vi "emi_FP Show.vi"(5 "VI Refnum(This vi)":refnum<vi>, 7 "Show time s(0)":dbl, 9 "error in (no error)":errorcluster) -> (6 "VI Refnum":refnum<vi>, 10 "error out":errorcluster)   [LabVIEW 2011]
doc: "If Front panel not open, opens it\nFades in 'vi to tarnsparensy = 0%\nUses time instead of number of iterations to avoid overly long fade ins when processing power is at a premium.\ns\nIf no VI ref in, then the VI containing this VI is used.\nIf VI has multiple panes, only the first pane will be used.\n\nOn error in: Does not run."
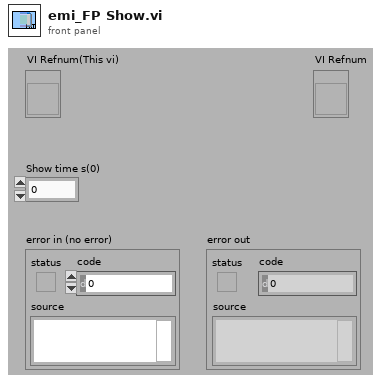
[diagram p1: front panel]
types:
  T1 = enum32{"Invalid", "Standard", "Closed", "Hidden", "Minimized", "Maximized"}
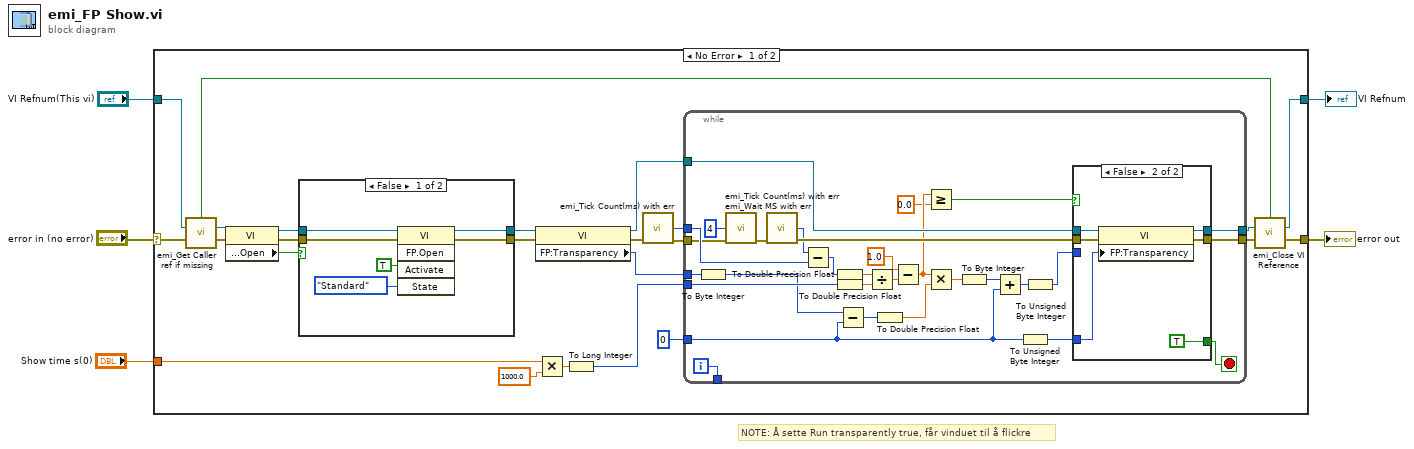
[diagram p0: block diagram]
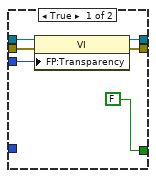
[diagram p3: hidden frame]
diagram:
  # "NOTE: Å sette Run transparently true, får vinduet til å flickre"
  n1 = case shown="No Error" "error in (no error)" {
    selector: "error in (no error)" -> [w28 w81]
    tunnel: [w26 w81] -> w5
    tunnel: "VI Refnum(This vi)" -> [w27 w80]
    tunnel: [w25 w80] -> w3
    tunnel: "Show time s(0)" -> [w19 _]
    frame No Error {
      n2 = call "emi_Get Caller ref if missing.vi"("VI Refnum(Calling VI)"=w27, "error in (no error)"=w28) -> ("Ref Generated"=w29:bool, "VI Refnum Out"=w11:refnum<vi>, "error out"=w12:errorcluster)  [unwired: 11 in]
      n3 = property class="VI"(reference=w11, error in=w12) -> (reference out=w8:refnum<vi>, error out=w9:errorcluster, "Front Panel.Open"=w10:bool)
      n4 = case shown="False" w10 {
        tunnel: w9 -> [w34 w36]
        tunnel: w8 -> [w35 w37]
        tunnel: [w33 w36] -> w7
        tunnel: [w32 w37] -> w6
        frame False {
          n5 = invoke class="VI" method="FP.Open"(reference=w35, error in=w34, "Activate"=TRUE ("Activate?"), "State"=T1."Standard") -> (reference out=w32:refnum<vi>, error out=w33:errorcluster)  [unwired: 1 in, 3 out]
        }
        frame True {
        }
      }
      n6 = property class="VI"(reference=w6, error in=w7) -> (reference out=w22:refnum<vi>, error out=w24:errorcluster, "FP:Transparency"=w20:u8)
      n7 = Multiply(x=w19, y=1000.0) -> (x*y=w17:dbl)
      n8 = To Long Integer(number=w17) -> (32bit integer=w16:i32)
      n9 = call "emi_Tick Count(ms) with err.vi"("error in (no error)"=w24) -> ("millisecond timer value"=w21:u32, "error out"=w23:errorcluster)  [unwired: 13 in]
      n10 = while {
        tunnel: w23 -> [w61]
        tunnel: w22 -> [w65]
        tunnel: w21 -> [w62]
        tunnel: [w67] -> w14
        tunnel: [w64] -> w15
        tunnel: w20 -> [w45]
        tunnel: w16 -> [w57]
        tunnel: [w49] -> _
        tunnel: i8 0 ("Target Transparensy %(100)") -> [w38]
        i -> [w49]
        stop <- w50 stop-if-true
        n11 = To Byte Integer(number=w45) -> (8bit integer=w44:i8)
        n12 = call "emi_Wait MS with err.vi"("milliseconds to wait(0)"=u32 4, "error in (no error)"=w61) -> ("error out"=w60:errorcluster)  [unwired: 13 in]
        n13 = call "emi_Tick Count(ms) with err.vi"("error in (no error)"=w60) -> ("millisecond timer value"=w63:u32, "error out"=w66:errorcluster)  [unwired: 13 in]
        n14 = Subtract(x=w63, y=w62) -> (x-y=w58:u32)
        n15 = To Double Precision Float(number=w58) -> (double precision float=w56:dbl)
        n16 = To Double Precision Float(number=w57) -> (double precision float=w55:dbl)
        n17 = Subtract(x=w44, y=w38) -> (x-y=w46:i8)
        n18 = Divide(x=w56, y=w55) -> (x/y=w54:dbl)
        n19 = To Double Precision Float(number=w46) -> (double precision float=w48:dbl)
        n20 = Subtract(x=1.0, y=w54) -> (x-y=w41:dbl)
        n21 = Greater Or Equal?(x=w41, y=0.0) -> (x >= y?=w39:bool)
        n22 = Multiply(x=w41, y=w48) -> (x*y=w51:dbl)
        n23 = To Byte Integer(number=w51) -> (8bit integer=w52:i8)
        n24 = Add(x=w52, y=w38) -> (x+y=w47:i8)
        n25 = To Unsigned Byte Integer(number=w38) -> (unsigned 8bit integer=w42:u8)
        n26 = To Unsigned Byte Integer(number=w47) -> (unsigned 8bit integer=w43:u8)
        n27 = case shown="False" w39 {
          tunnel: [w73 w76] -> w67
          tunnel: w66 -> [w72 w78]
          tunnel: w65 -> [w71 w77]
          tunnel: [w70 w75] -> w64
          tunnel: [FALSE TRUE] -> w50
          tunnel: w42 -> [_ w74]
          tunnel: w43 -> [w68 _]
          frame True {
            n28 = property class="VI"(reference=w71, error in=w72, "FP:Transparency"=w68) -> (reference out=w70:refnum<vi>, error out=w73:errorcluster)
          }
          frame False {
            n29 = property class="VI"(reference=w77, error in=w78, "FP:Transparency"=w74) -> (reference out=w75:refnum<vi>, error out=w76:errorcluster)
          }
        }
      }
      n30 = call "emi_Close VI Reference.vi"("Close ref?(T)"=w29, "VI Refnum"=w15, "error in (no error)"=w14) -> ("VI Refnum Out"=w25:refnum<vi>, "error out"=w26:errorcluster)  [unwired: 11 in]
    }
    frame Error {
    }
  }
  "error out" <- w5
  "VI Refnum" <- w3
